vi "main.vi"(0 "File Path":path, 5 "Log to File":bool, 11 "Error In":errorcluster) -> (15 "Error Out":errorcluster)   [LabVIEW 2023]
doc: "This VI reads a text file containing file and folder paths, sorts them based on disk hierarchy in reverse alphabetical order, and displays the sorted paths with their sizes in a table. The results can be saved to a CSV file."
uses:
  Library/File Path Operations/Controls/Data.ctl
  <vilib>/Utility/error.llb/Trim Whitespace One-Sided.vi
  Library/File Path Operations/File and Path Operations.lvlib
panel:
  out "Table Control":string[][](table)
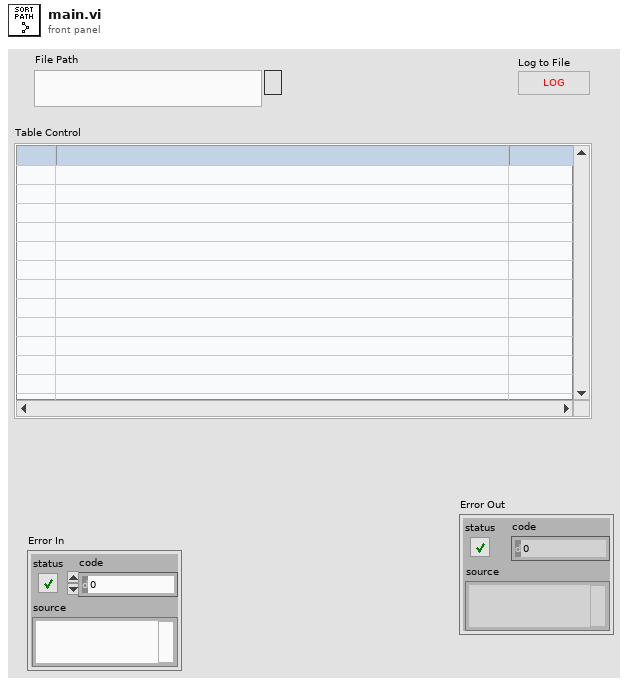
[diagram p1: front panel]
types:
  T1 = typedef "File and Path Operations.lvlib/Data.ctl" = cluster{"List of Paths":string[][], "Serial No":i32}
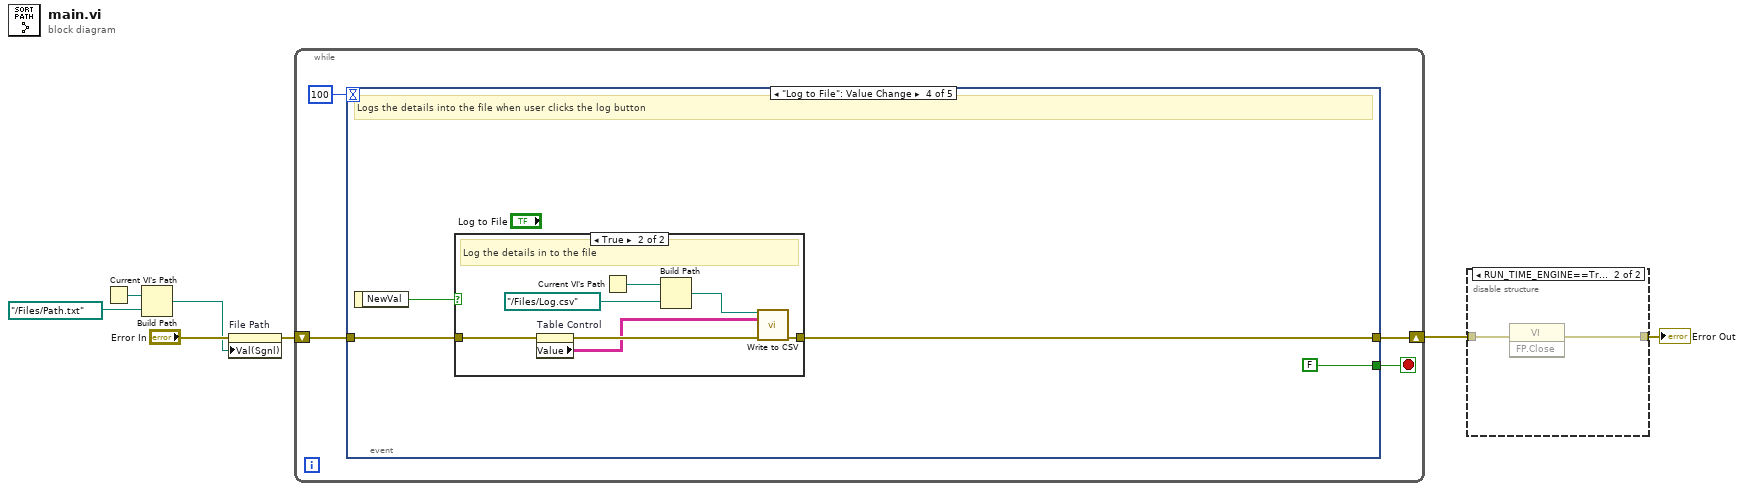
[diagram p0: block diagram]
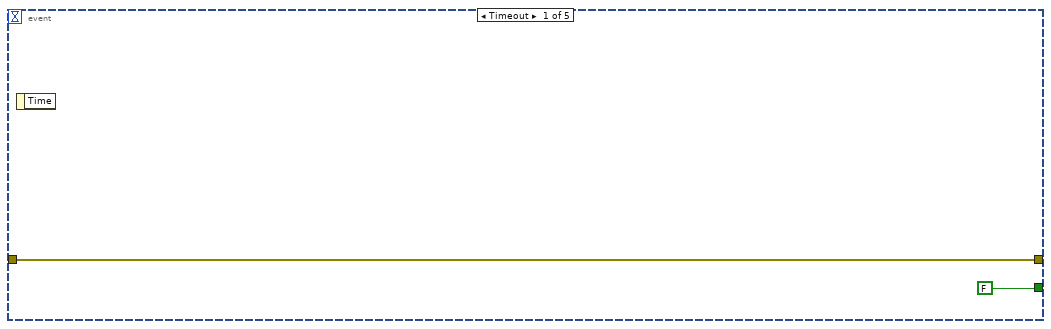
[diagram p3: hidden frame]
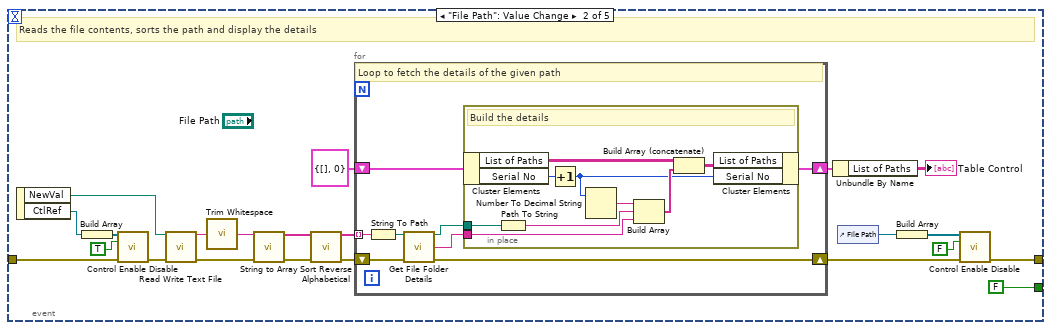
[diagram p4: hidden frame]
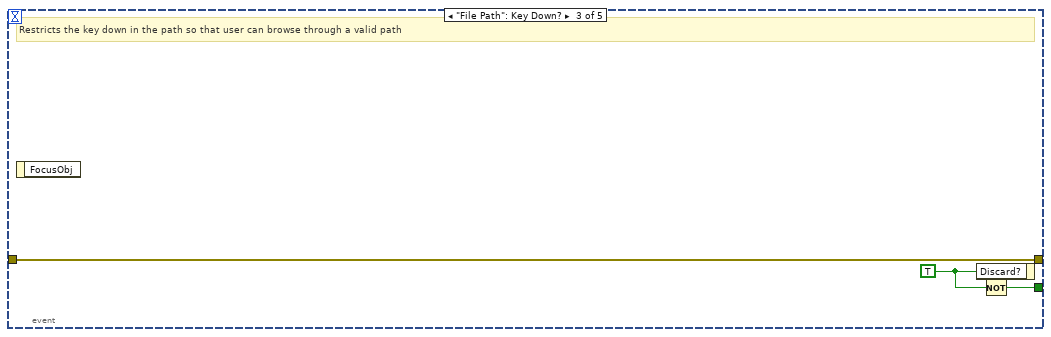
[diagram p5: hidden frame]
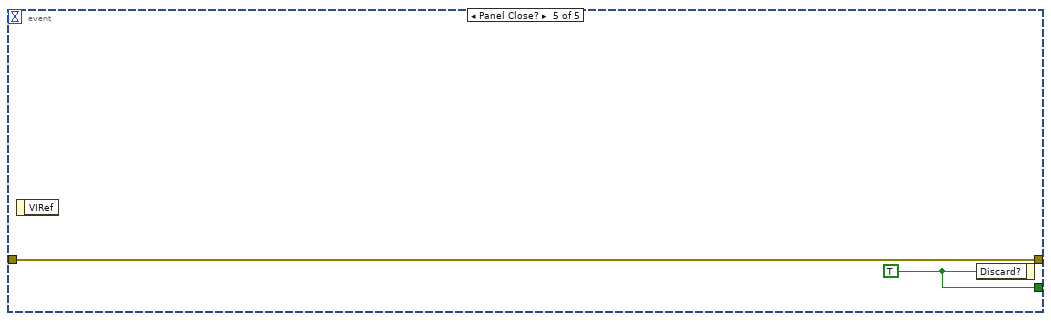
[diagram p7: hidden frame]
diagram:
  n1 = Current VI's Path() -> (path=w4:path)
  n2 = Build Path(base path=w4, name or relative path=path "../Files/Path.txt") -> (appended path=w2:path)
  n3 = property on="File Path" class="Path"(error in="Error In", "Val(Sgnl)"=w2) -> (error out=w5:errorcluster)  [unwired: 1 in, 1 out]
  n4 = while {
    shift-right: [w10] -> w6
    shift-left: w5 -> [w11]
    stop <- w8 stop-if-true
    n5 = event shown="[3] \"Log to File\": Value Change" {
      selector: _ -> [_ _ _ _ _]
      dyn-events: _ -> [_ _ _ _ _]
      timeout: 100 -> [_ _ _ _ _]
      tunnel: w11 -> [w13 w35 w55 w59 w69]
      tunnel: [w13 w15 w55 w58 w69] -> w10
      tunnel: [FALSE FALSE w53 FALSE w68] -> w8
      event Timeout {
        n6 = event-data() -> ()  [unwired: 1 in, 1 out]
      }
      event "File Path": Value Change {
        # "Reads the file contents, sorts the path and display the details"
        n7 = event-data() -> ("NewVal"=w25:path, "CtlRef"=w21:refnum<vi>)  [unwired: 1 in]
        n8 = Build Array(w21) -> (w20:refnum<vi>[])
        n9 = call "Control Enable Disable.vi"("Control References"=w20, "Disable?"=TRUE, "Error In"=w35) -> ("Error Out"=w22:errorcluster)  [unwired: 12 in]
        n10 = call "Read Write Text File.vi"("File Path"=w25, "Error In"=w22) -> ("Text Output"=w34:string, "Error Out"=w33:errorcluster)  [unwired: 12 in]
        n11 = call <vilib>:"Trim Whitespace.vi"("string"=w34) -> ("trimmed string"=w23:string)  [unwired: 1 in]
        n12 = call "String to Array.vi"("Input String"=w23, "Error In"=w33) -> ("Array of Strings"=w31:string[], "Error Out"=w32:errorcluster)  [unwired: 12 in]
        n13 = call "Sort Reverse Alphabetical.vi"("Unsorted Array"=w31, "Error In"=w32) -> ("Sorted Array"=w29:string[], "Error Out"=w30:errorcluster)  [unwired: 12 in]
        n14 = for {
          shift-right: [w42] -> w16
          shift-left: w30 -> [w43]
          tunnel: w29 -> [w41] mode=indexing
          shift-right: [w37] -> w27
          shift-left: T1 {"List of Paths"=[], "Serial No"=0} -> [w38]
          # "Loop to fetch the details of the given path"
          n15 = String To Path(string=w41) -> (path=w40:path)
          n16 = call "Get File Folder Details.vi"("Path"=w40, "Error In"=w43) -> ("Parent Path"=w36:path, "Size"=w39:string, "Error Out"=w42:errorcluster)  [unwired: 10 in, 1 out]
          n17 = in-place {
            in-place-border: w39 -> [w49]
            in-place-border: w36 -> [w45]
            # "Build the details"
            n18 = in-place-cluster #1(w38) -> ("List of Paths"=w46:string[][], "Serial No"=w50:i32)
            n19 = Path To String(path=w45) -> (string=w44:string)
            n20 = Increment(x=w50) -> (x+1=w47:i32)
            n21 = Number To Decimal String(number=w47) -> (decimal integer string=w52:string)  [unwired: 1 in]
            n22 = Build Array(w52, w44, w49) -> (w51:string[])
            n23 = Build Array (concatenate)(w46, w51) -> (w48:string[][])
            n24 = in-place-cluster #1("List of Paths"=w48, "Serial No"=w47) -> (w37:T1)
          }
        }
        n25 = Unbundle By Name(w27) -> ("List of Paths"=→"Table Control":string[][])
        n26 = control-ref of="File Path"() -> (w14:refnum<vi>)
        n27 = Build Array(w14) -> (w18:refnum<vi>[])
        n28 = call "Control Enable Disable.vi"("Control References"=w18, "Disable?"=FALSE, "Error In"=w16) -> ("Error Out"=w15:errorcluster)  [unwired: 12 in]
      }
      event "File Path": Key Down? {
        w54 = TRUE ("Discard?")
        # "Restricts the key down in the path so that user can browse through a valid path"
        n29 = event-data() -> ()  [unwired: 1 in, 1 out]
        n30 = event-data("Discard?"=w54) -> ()  [unwired: 1 in, 1 out]
        n31 = Not(x=w54) -> (.not. x?=w53:bool)
      }
      event "Log to File": Value Change {
        # "Logs the details into the file when user clicks the log button"
        n32 = event-data() -> ("NewVal"=w57:bool)  [unwired: 1 in]
        n33 = case shown="True" w57 {
          tunnel: w59 -> [w60 w66]
          tunnel: [w60 w67] -> w58
          frame False {
          }
          frame True {
            # "Log the details in to the file"
            n34 = property on="Table Control" class="Tbl (strict)"(error in=w66) -> (error out=w65:errorcluster, "Value"=w64:string[][])  [unwired: 1 in, 1 out]
            n35 = Current VI's Path() -> (path=w63:path)
            n36 = Build Path(base path=w63, name or relative path=path "../Files/Log.csv") -> (appended path=w61:path)
            n37 = call "Write to CSV.vi"("Path In"=w61, "Array In"=w64, "Error In"=w65) -> ("Error Out"=w67:errorcluster)  [unwired: 10 in, 2 out]
          }
        }
      }
      event Panel Close? {
        w68 = TRUE ("Discard?")
        n38 = event-data() -> ()  [unwired: 1 in, 1 out]
        n39 = event-data("Discard?"=w68) -> ()  [unwired: 1 in, 1 out]
      }
    }
  }
  n40 = disable-structure shown="RUN_TIME_ENGINE==True" {
    disable-tunnel: w6 -> [w70 w72]
    disable-tunnel: [w70 w71] -> w1
    frame condition #0 (active) {
    }
    frame condition #1 {
      n41 = invoke class="VI" method="FP.Close"(error in=w72) -> (error out=w71:errorcluster)  [unwired: 2 in, 2 out]
    }
  }
  "Error Out" <- w1
